vi "checkDO.vi"(6 "expect tangent":dbl, 7 "times":u16, 8 "down":dbl, 9 "up":dbl, 10 "sample sn":string[](array[string]), 11 "sample port":refnum<visa-resource-name>[](array[refnum])) -> (0 "DO":string[](array[string]), 1 "ok":bool, 2 "Array":bool[](array[boolean]))   [LabVIEW 2012]
uses:
  globalstatus.vi
panel:
  out "DO pool":dbl[][](array[numeric])
  out "count":u16
  in  "Enum":enum16{"excit", "get tangent"}(ring)
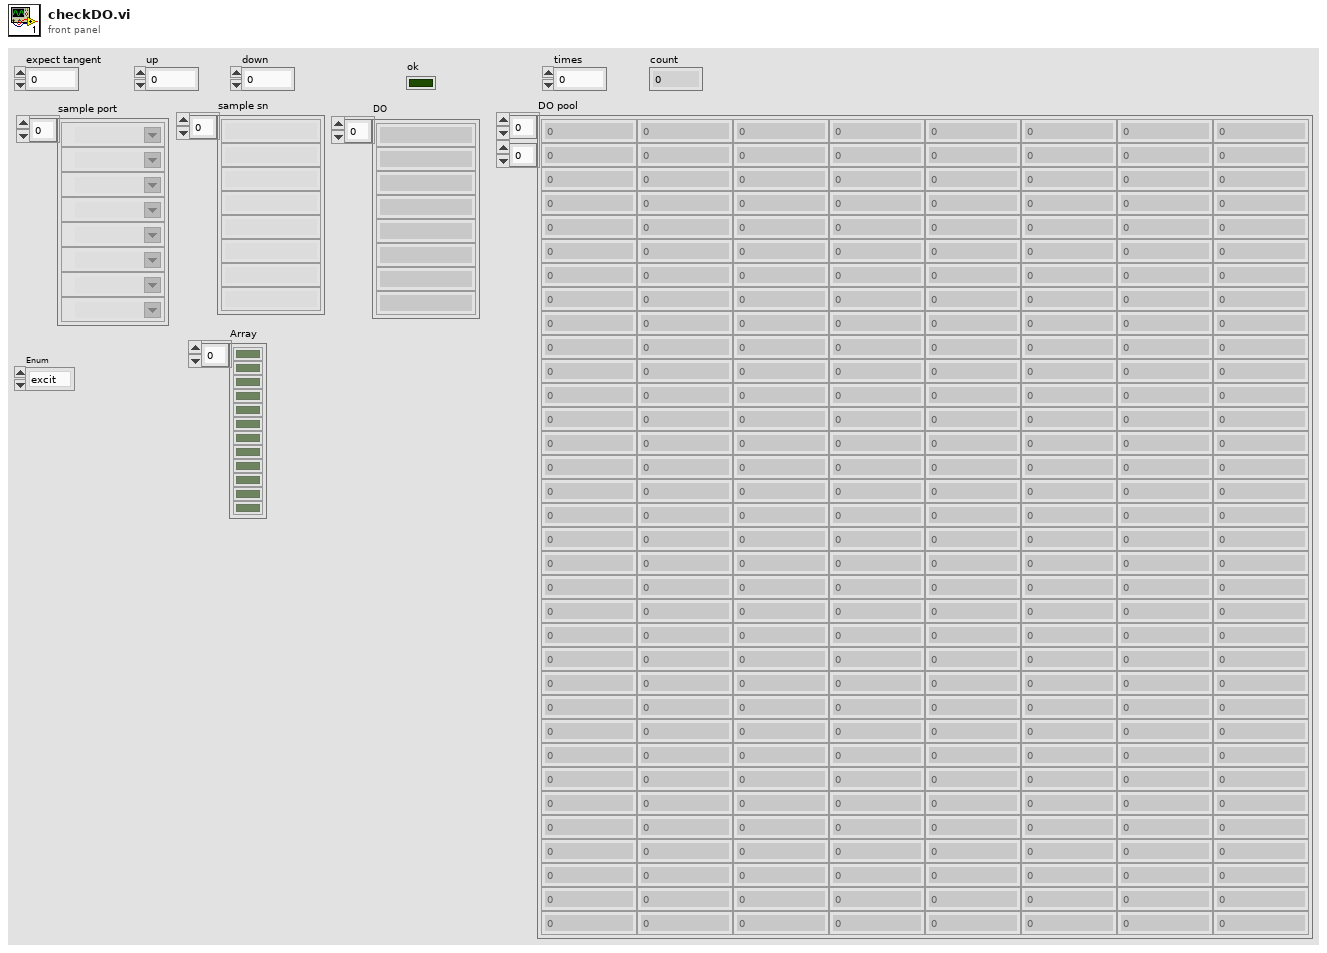
[diagram p1: front panel]
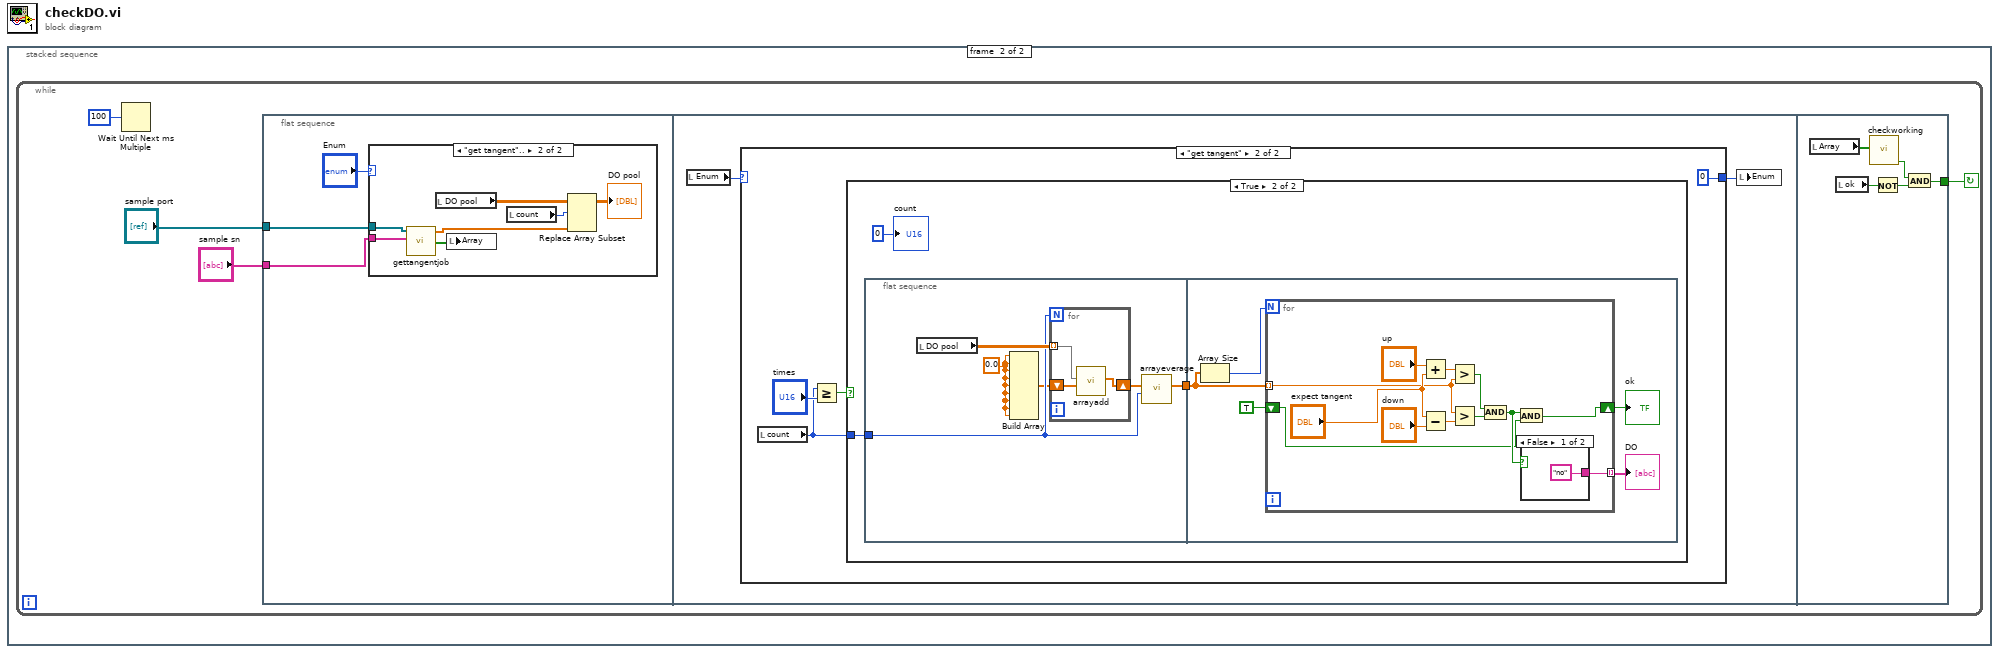
[diagram p0: block diagram]
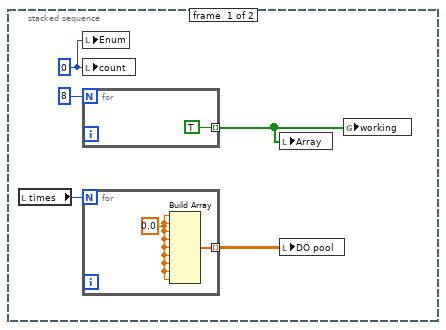
[diagram p2: hidden frame]
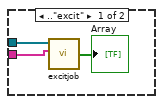
[diagram p3: hidden frame]
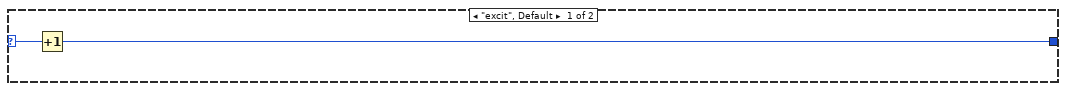
[diagram p4: hidden frame]
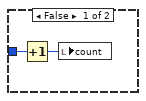
[diagram p5: hidden frame]
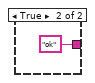
[diagram p6: hidden frame]
diagram:
  n1 = stacked-sequence {
    frame #0 {
      w3 = 0
      n2 = local read "times"() -> (w5:u16)
      n3 = local write "Enum"(w3) -> ()
      n4 = local write "count"(w3) -> ()
      n5 = for {
        N: 8 -> [_]
        tunnel: [TRUE] -> w1 mode=indexing
      }
      n6 = for {
        N: w5 -> [_]
        tunnel: [w7] -> w4 mode=indexing
        w8 = 0.0
        n7 = Build Array(w8, w8, w8, w8, w8, w8, w8, w8, w8) -> (w7:dbl[])
      }
      n8 = local write "Array"(w1) -> ()
      n9 = local write "DO pool"(w4) -> ()
      n10 = global write "globalstatus.vi" "working"(w1) -> ()
    }
    frame #1 {
      n11 = while {
        stop <- w9 continue-if-true
        n12 = Wait Until Next ms Multiple(millisecond multiple=100) -> ()  [unwired: 1 out]
        n13 = flat-sequence {
          tunnel: "sample port" -> [w15]
          tunnel: "sample sn" -> [w14]
          tunnel: [w69] -> w9
          frame #0 {
            n14 = case shown="\"get tangent\".." "Enum" {
              tunnel: w15 -> [w18 w25]
              tunnel: w14 -> [w17 w24]
              frame .."excit" {
                n15 = call "excitjob.vi"("sample port"=w18, "sample sn"=w17) -> ("Array"=→"Array":bool[])  [unwired: 5 in, 1 out]
              }
              frame "get tangent".. {
                n16 = call "gettangentjob.vi"("sample port"=w25, "sample sn"=w24) -> ("tangent"=w21:dbl[], "Array"=w23:bool[])  [unwired: 5 in]
                n17 = local read "DO pool"() -> (w22:dbl[][])
                n18 = local write "Array"(w23) -> ()
                n19 = local read "count"() -> (w20:u16)
                n20 = Replace Array Subset(array=w22, new element=w21, index (row)=w20) -> (→"DO pool":dbl[][])  [unwired: 1 in]
              }
            }
          }
          frame #1 {
            n21 = local read "Enum"() -> (w27:enum16{"excit", "get tangent"})
            n22 = case shown="\"get tangent\"" w27 {
              selector: w27 -> [w29 _]
              tunnel: [w28 0] -> w26
              frame "excit", Default {
                n23 = Increment(x=w29) -> (x+1=w28:enum16{"excit", "get tangent"})
              }
              frame "get tangent" {
                n24 = local read "count"() -> (w30:u16)
                n25 = Greater Or Equal?(x=w30, y="times") -> (x >= y?=w32:bool)
                n26 = case shown="True" w32 {
                  tunnel: w30 -> [w35 w37]
                  frame False {
                    n27 = Increment(x=w35) -> (x+1=w34:u16)
                    n28 = local write "count"(w34) -> ()
                  }
                  frame True {
                    n29 = flat-sequence {
                      tunnel: w37 -> [w42]
                      tunnel: [w41] -> w36
                      tunnel: w36 -> [w51]
                      frame #0 {
                        w40 = 0.0
                        n30 = local read "DO pool"() -> (w44:dbl[][])
                        n31 = Build Array(w40, w40, w40, w40, w40, w40, w40, w40, w40) -> (w39:dbl[])
                        n32 = for {
                          N: w42 -> [_]
                          tunnel: w44 -> [w47] mode=indexing
                          shift-right: [w46] -> w43
                          shift-left: w39 -> [w45]
                          n33 = call "arrayadd.vi"("b"=w45, "a"=w47) -> ("c"=w46:dbl[])  [unwired: 9 in]
                        }
                        n34 = call "arrayeverage.vi"("divider"=w42, "in"=w43) -> ("out"=w41:dbl[])  [unwired: 9 in]
                      }
                      frame #1 {
                        n35 = Array Size(array=w51) -> (size(s)=w52:i32)
                        n36 = for {
                          N: w52 -> [_]
                          tunnel: w51 -> [w59] mode=indexing
                          shift-right: [w55] -> w49
                          shift-left: TRUE -> [w54]
                          tunnel: [w53] -> w48 mode=indexing
                          n37 = Add(x="up", y="expect tangent") -> (x+y=w60:dbl)
                          n38 = Subtract(x="expect tangent", y="down") -> (x-y=w61:dbl)
                          n39 = Greater?(x=w60, y=w59) -> (0:w57:bool)
                          n40 = Greater?(x=w59, y=w61) -> (0:w58:bool)
                          n41 = And(x=w57, y=w58) -> (x .and. y?=w56:bool)
                          n42 = And(x=w56, y=w54) -> (x .and. y?=w55:bool)
                          n43 = case shown="False" w56 {
                            tunnel: ["no" "ok"] -> w53
                            frame False {
                            }
                            frame True {
                            }
                          }
                        }
                        "ok" <- w49
                        "DO" <- w48
                      }
                    }
                    "count" <- 0
                  }
                }
              }
            }
            n44 = local write "Enum"(w26) -> ()
          }
          frame #2 {
            n45 = local read "Array"() -> (w71:bool[])
            n46 = local read "ok"() -> (w68:bool)
            n47 = call "checkworking.vi"("Array"=w71) -> ("Boolean"=w70:bool)  [unwired: 8 in]
            n48 = Not(x=w68) -> (.not. x?=w67:bool)
            n49 = And(x=w70, y=w67) -> (x .and. y?=w69:bool)
          }
        }
      }
    }
  }
